vi "wmf_list_cameras.vi"(8 "error in (no error)":errorcluster) -> (0 "error out":errorcluster, 2 "Modes":T1(array[cluster]), 3 "Cam Names":string[](array[string]))   [LabVIEW 2022 SP3, in "Vision.lvlib"]
uses:
  Vision.lvlib
  bin/Camera.dll
panel:
  out "size(s)":i32[](array[numeric])
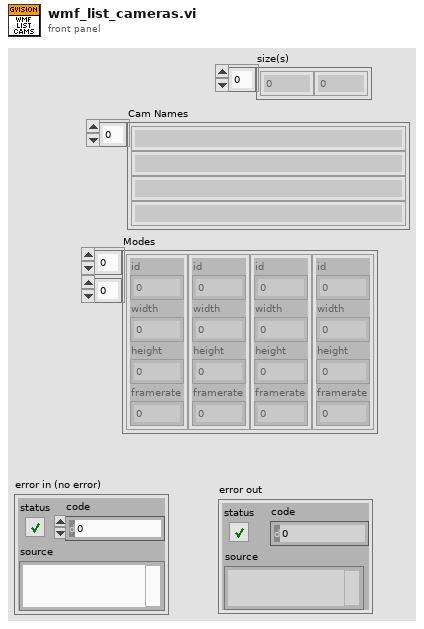
[diagram p1: front panel]
types:
  T1 = cluster{"id":i32, "width":i32, "height":i32, "framerate":sgl}[][]
  T2 = cluster{"id":i32, "width":i32, "height":i32, "framerate":sgl}[]
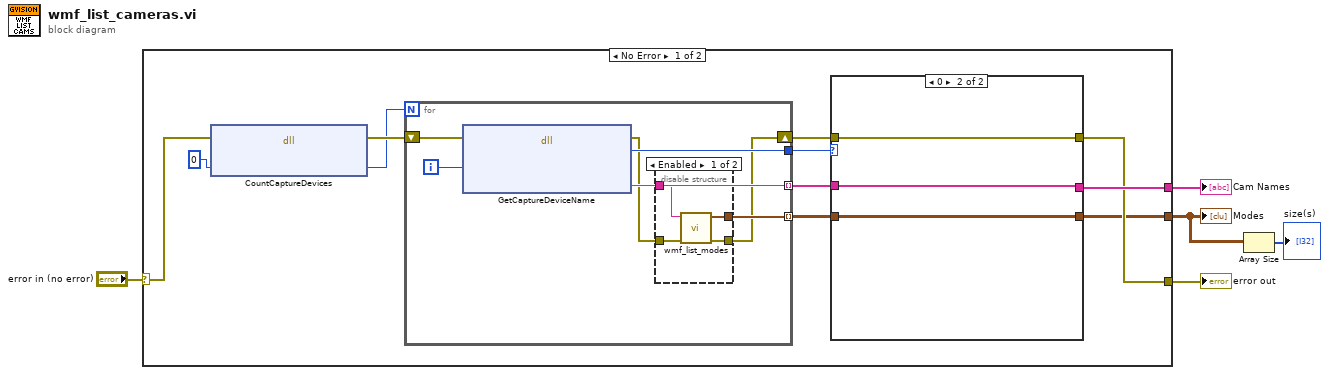
[diagram p0: block diagram]
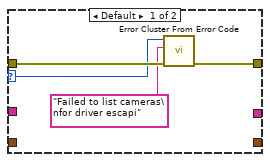
[diagram p3: hidden frame]
diagram:
  n1 = case shown="No Error" "error in (no error)" {
    selector: "error in (no error)" -> [w16 w35]
    tunnel: [w13 w35] -> w4
    tunnel: [w14 _] -> w3
    tunnel: [w6 _] -> w2
    frame No Error {
      n2 = dll-call lib="C:/Users/Caleb/Desktop/nebraska-silicon-lab/pixel-gantry-extra/LV/bin/Camera.dll" fn="CountCaptureDevices"(error in=w16, "count"=0 ("n_cameras")) -> (error out=w12:errorcluster, "count"=w9:i32)  [unwired: 3 in, 1 out]
      n3 = for {
        N: w9 -> [_]
        shift-right: [w17] -> w10
        shift-left: w12 -> [w22]
        tunnel: [w21] -> w11
        tunnel: [w20] -> w8 mode=indexing
        tunnel: [w18] -> w7 mode=indexing
        i -> [w23]
        n4 = dll-call lib="C:/Users/Caleb/Desktop/nebraska-silicon-lab/pixel-gantry-extra/LV/bin/Camera.dll" fn="GetCaptureDeviceName"(error in=w22, "camera_id"=w23) -> (error out=w19:errorcluster, "return type"=w21:i32, "name_lsh"=w20:string)  [unwired: 4 in, 1 out]
        n5 = disable-structure shown="Enabled" {
          disable-tunnel: w20 -> [w27 _]
          disable-tunnel: w19 -> [w26 _]
          disable-tunnel: [w25 _] -> w18
          disable-tunnel: [w24 _] -> w17
          frame Enabled {
            n6 = call "wmf_list_modes.vi"("error in (no error)"=w26, "camera_name"=w27) -> ("error out"=w24:errorcluster, "Modes"=w25:T2)  [unwired: 8 in]
          }
          frame Disabled {
          }
        }
      }
      n7 = case shown="0" w11 {
        selector: w11 -> [w29 _]
        tunnel: [_ w33] -> w14
        tunnel: w10 -> [w31 w34]
        tunnel: [w30 w34] -> w13
        tunnel: w8 -> [_ w33]
        tunnel: w7 -> [_ w32]
        tunnel: [_ w32] -> w6
        frame Default {
          n8 = call <vilib>:"Error Cluster From Error Code.vi"("error in (no error)"=w31, "error message (\"\")"="Failed to list cameras\nfor driver escapi" ("error message (\"\")"), "error code (0)"=w29) -> ("error out"=w30:errorcluster)  [unwired: 6 in]
        }
        frame 0 {
        }
      }
    }
    frame Error {
    }
  }
  "error out" <- w4
  "Cam Names" <- w3
  "Modes" <- w2
  n9 = Array Size(array=w2) -> (size(s)=→"size(s)":i32[])
